vi "Stop Acquisition.vi"(8 "error in (no error)":errorcluster, 11 "Hardware Resources in":T1={"AI"={"task name"="", "task_ref"="", "physical channels"="Dev1/ai0:7", "channels config"={"input terminal configuration"=0, "minimum value"=-5.0, "maximum value"=5.0}, "rate"=1000.0}, "conversions"={"ai0"={"a"=0.0, "b"=0.0}, "ai1"={"a"=0.0, "b"=0.0}, "ai2"={"a"=0.0, "b"=0.0}, "ai3"={"a"=0.0, "b"=0.0}, "ai4"={"a"=0.0, "b"=0.0}}, "compteur 0"={"task name"="CTR", "task_ref"="", "ctr"="Dev1/ctr0:3", "coeff"=4000.0}, "compteur 1"={"task name"="CTR1", "task_ref"="", "ctr"="Dev1/ctr1", "coeff"=4000.0}, "compteur 2"={"task name"="CTR2", "task_ref"="", "ctr"="Dev1/ctr2", "coeff"=4000.0}, "compteur 3"={"task name"="CTR3", "task_ref"="", "ctr"="Dev1/ctr3", "coeff"=4000.0}} {"compteur 3"."coeff" format="%0.2f"; "compteur 2"."coeff" format="%0.2f"; "compteur 1"."coeff" format="%0.2f"; "compteur 0"."coeff" format="%0.2f"; "AI"."rate" format="%0.2f"; "AI"."channels config"."input terminal configuration" items=["Default"=-1, "RSE"=10083, "NRSE"=10078, "Differential"=10106, "Pseudodifferential"=12529]}) -> (0 "error out":errorcluster)   [LabVIEW 2014, in "PLS Acquisition.lvlib"]
doc: "Stops the acquisition."
uses:
  PLS Acquisition.lvlib
  Hardware Configuration.ctl
  Settings/conversion.ctl
  Settings/PLS Settings.lvlib
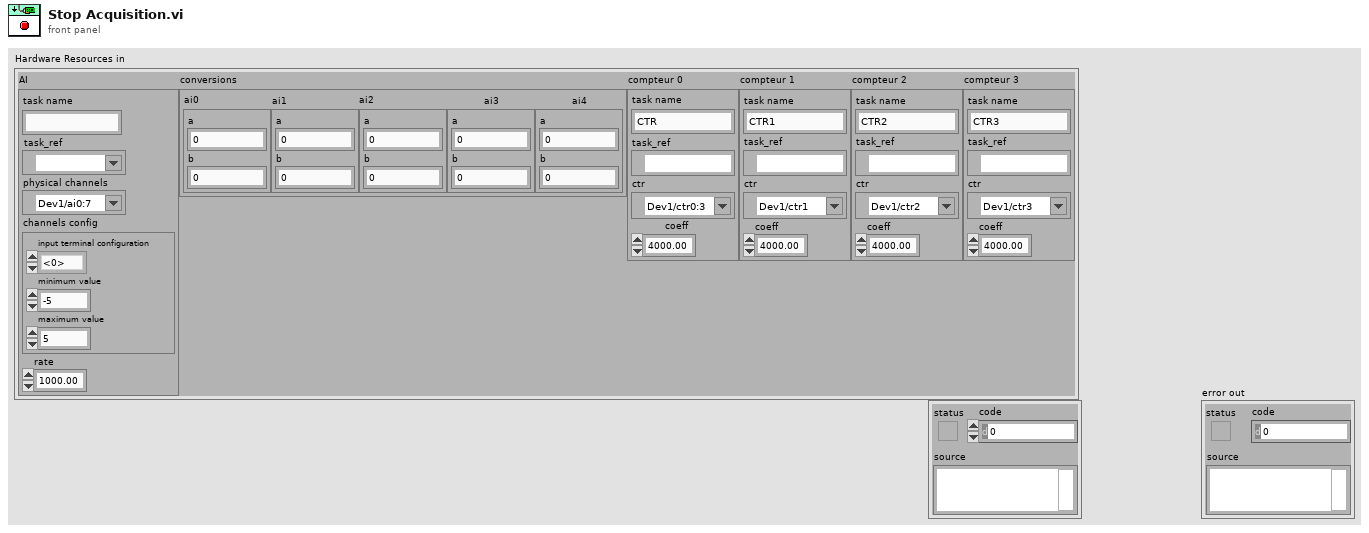
[diagram p1: front panel]
types:
  T1 = typedef "PLS Acquisition.lvlib/Hardware Configuration.ctl" = cluster{"AI":cluster{"task name":string, "task_ref":refnum<k21>, "physical channels":tag, "channels config":cluster{"input terminal configuration":i32, "minimum value":dbl, "maximum value":dbl}, "rate":dbl}, "conversions":cluster{"ai0":T2, "ai1":T2, "ai2":T2, "ai3":T2, "ai4":T2}, "compteur 0":cluster{"task name":string, "task_ref":refnum<k21>, "ctr":tag, "coeff":dbl}, "compteur 1":cluster{"task name":string, "task_ref":refnum<k21>, "ctr":tag, "coeff":dbl}, "compteur 2":cluster{"task name":string, "task_ref":refnum<k21>, "ctr":tag, "coeff":dbl}, "compteur 3":cluster{"task name":string, "task_ref":refnum<k21>, "ctr":tag, "coeff":dbl}}
  T2 = typedef "PLS Settings.lvlib/conversion.ctl" = cluster{"a":dbl, "b":dbl}
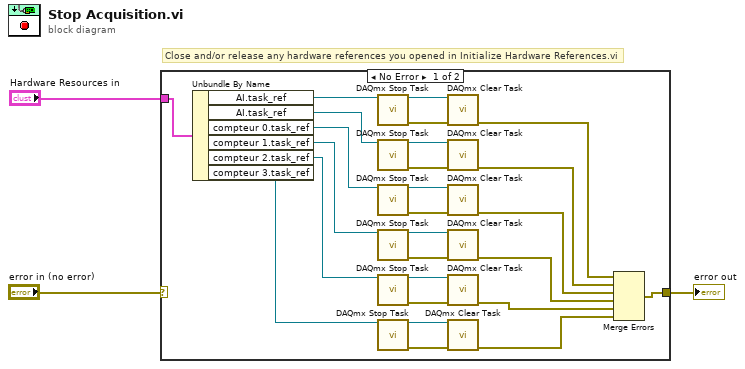
[diagram p0: block diagram]
diagram:
  # "Close and/or release any hardware references you opened in Initialize Hardware References.vi"
  n1 = case shown="No Error" "error in (no error)" {
    selector: "error in (no error)" -> [_ w30]
    tunnel: [w29 w30] -> w2
    tunnel: "Hardware Resources in" -> [w28 _]
    frame No Error {
      n2 = Unbundle By Name(w28) -> ("AI.task_ref"=w27:refnum<k21>, "AI.task_ref"=w18:refnum<k21>, "compteur 0.task_ref"=w12:refnum<k21>, "compteur 1.task_ref"=w11:refnum<k21>, "compteur 2.task_ref"=w10:refnum<k21>, "compteur 3.task_ref"=w9:refnum<k21>)
      n3 = call <vilib>:"DAQmx Stop Task.vi"("task/channels in"=w27) -> ("task out"=w26:refnum<k21>, "error out"=w25:errorcluster)  [unwired: 13 in]
      n4 = call <vilib>:"DAQmx Stop Task.vi"("task/channels in"=w18) -> ("task out"=w17:refnum<k21>, "error out"=w23:errorcluster)  [unwired: 13 in]
      n5 = call <vilib>:"DAQmx Stop Task.vi"("task/channels in"=w12) -> ("task out"=w16:refnum<k21>, "error out"=w21:errorcluster)  [unwired: 13 in]
      n6 = call <vilib>:"DAQmx Stop Task.vi"("task/channels in"=w11) -> ("task out"=w15:refnum<k21>, "error out"=w22:errorcluster)  [unwired: 13 in]
      n7 = call <vilib>:"DAQmx Stop Task.vi"("task/channels in"=w10) -> ("task out"=w14:refnum<k21>, "error out"=w20:errorcluster)  [unwired: 13 in]
      n8 = call <vilib>:"DAQmx Stop Task.vi"("task/channels in"=w9) -> ("task out"=w13:refnum<k21>, "error out"=w19:errorcluster)  [unwired: 13 in]
      n9 = call <vilib>:"DAQmx Clear Task.vi"("task in"=w26, "error in"=w25) -> ("error out"=w24:errorcluster)  [unwired: 13 in]
      n10 = call <vilib>:"DAQmx Clear Task.vi"("task in"=w17, "error in"=w23) -> ("error out"=w8:errorcluster)  [unwired: 13 in]
      n11 = call <vilib>:"DAQmx Clear Task.vi"("task in"=w16, "error in"=w21) -> ("error out"=w7:errorcluster)  [unwired: 13 in]
      n12 = call <vilib>:"DAQmx Clear Task.vi"("task in"=w15, "error in"=w22) -> ("error out"=w6:errorcluster)  [unwired: 13 in]
      n13 = call <vilib>:"DAQmx Clear Task.vi"("task in"=w14, "error in"=w20) -> ("error out"=w5:errorcluster)  [unwired: 13 in]
      n14 = call <vilib>:"DAQmx Clear Task.vi"("task in"=w13, "error in"=w19) -> ("error out"=w4:errorcluster)  [unwired: 13 in]
      n15 = Merge Errors(w24, w8, w7, w6, w5, w4) -> (w29:errorcluster)
    }
    frame Error {
    }
  }
  "error out" <- w2
